vi "Send HELLO.vi"(10 "error in (no error)":errorcluster, 11 "WAMP Client in":refnum<class "WAMP Client.lvclass">) -> (2 "error out":errorcluster, 3 "WAMP Client out":refnum<class "WAMP Client.lvclass">)   [LabVIEW 2020, in "wamplv.lvlib" / "WAMP Client.lvclass"]
uses:
  WAMP Client.lvclass
  WAMP Client.lvclass/WAMP Client.ctl
  Comm Handlers/ICommHandler/ICommHandler.lvclass
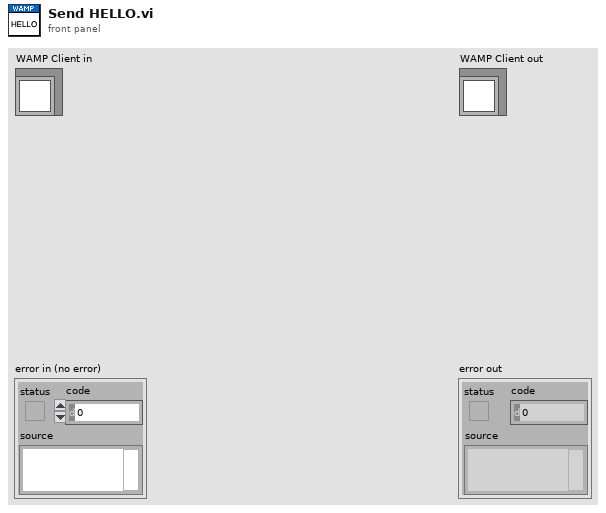
[diagram p1: front panel]
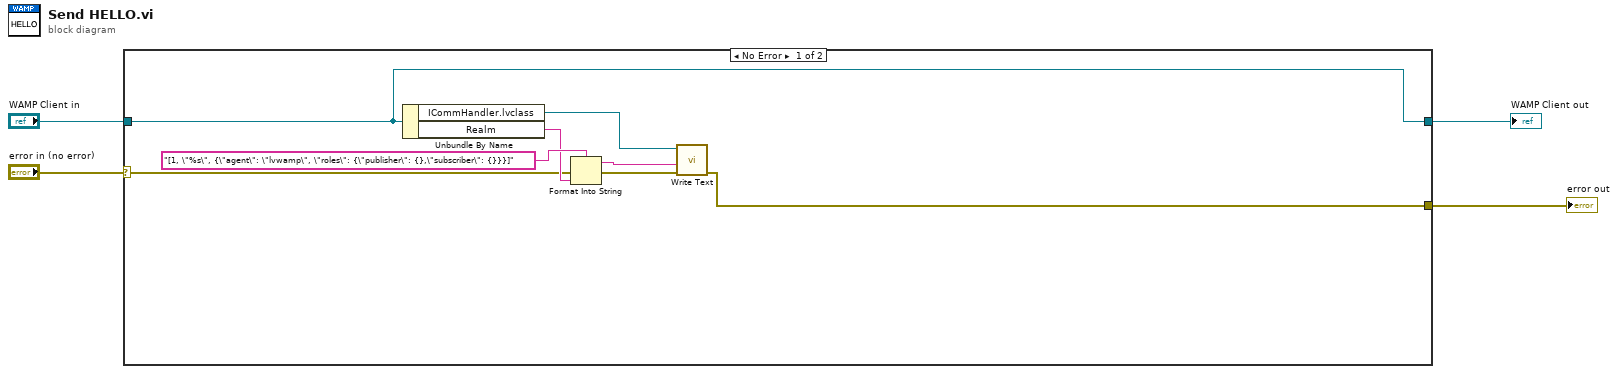
[diagram p0: block diagram]
diagram:
  n1 = case shown="No Error" "error in (no error)" {
    selector: "error in (no error)" -> [w7 w14]
    tunnel: [w5 w14] -> w3
    tunnel: [w11 w13] -> w1
    tunnel: "WAMP Client in" -> [w11 w13]
    frame No Error {
      n2 = Unbundle By Name(w11) -> ("ICommHandler.lvclass"=w12:refnum<class "ICommHandler.lvclass">, "Realm"=w9:string)
      n3 = Format Into String(format string="[1, \"%s\", {\"agent\": \"lvwamp\", \"roles\": {\"publisher\": {},\"subscriber\": {}}}]", error in=w7, w9) -> (resulting string=w8:string, error out=w6:errorcluster)  [unwired: 1 in]
      n4 = call-dynamic "Write Text.vi"("error in (no error)"=w6, "String"=w8, "ICommHandler in"=w12) -> ("error out"=w5:errorcluster)  [unwired: 7 in, 1 out]
    }
    frame Error {
    }
  }
  "error out" <- w3
  "WAMP Client out" <- w1
